vi "исходные пределы.vi"() -> ()   [LabVIEW 2013]
panel:
  in  "X1":dbl[][](array[numeric])=[[0.1, 20.0], [0.5, 200.0], [1.0, 200.0], [3.0, 2000.0], [5.0, 2000.0], [10.0, 2000.0], [15.0, 10000.0], [20.0, 10000.0], [25.0, 10000.0], [30.0, 10000.0], [35.0, 10000.0], [40.0, 10000.0], [45.0, 10000.0], [50.0, 10000.0], [55.0, 10000.0], [60.0, 10000.0], [65.0, 10000.0], [70.0, 10000.0], [75.0, 10000.0], [80.0, 10000.0], [85.0, 10000.0], [90.0, 10000.0], [95.0, 10000.0], [100.0, 10000.0]] format="%0.3f"
  in  "X2":dbl[][](array[numeric])=[[0.1, 20.0], [0.5, 200.0], [1.0, 200.0], [3.0, 200.0], [5.0, 2000.0], [10.0, 2000.0], [15.0, 2000.0], [20.0, 2000.0], [25.0, 2000.0], [30.0, 2000.0], [35.0, 2000.0], [40.0, 2000.0], [45.0, 10000.0], [50.0, 10000.0], [55.0, 10000.0], [60.0, 10000.0], [65.0, 10000.0], [70.0, 10000.0], [75.0, 10000.0], [80.0, 10000.0], [85.0, 10000.0], [90.0, 10000.0], [95.0, 10000.0], [100.0, 10000.0]] format="%0.3f"
  in  "X3":dbl[][](array[numeric])=[[0.1, 20.0], [0.5, 20.0], [1.0, 200.0], [3.0, 200.0], [5.0, 200.0], [10.0, 2000.0], [15.0, 2000.0], [20.0, 2000.0], [25.0, 2000.0], [30.0, 2000.0], [35.0, 2000.0], [40.0, 2000.0], [45.0, 2000.0], [50.0, 2000.0], [55.0, 2000.0], [60.0, 2000.0], [65.0, 2000.0], [70.0, 2000.0], [75.0, 2000.0], [80.0, 2000.0], [85.0, 2000.0], [90.0, 2000.0], [95.0, 2000.0], [100.0, 2000.0]] format="%0.3f"
  in  "X6":dbl[][](array[numeric])=[[0.1, 2.0], [0.5, 20.0], [1.0, 20.0], [3.0, 20.0], [5.0, 200.0], [10.0, 200.0], [15.0, 200.0], [20.0, 200.0], [25.0, 200.0], [30.0, 200.0], [35.0, 200.0], [40.0, 200.0], [45.0, 2000.0], [50.0, 2000.0], [55.0, 2000.0], [60.0, 2000.0], [65.0, 2000.0], [70.0, 2000.0], [75.0, 2000.0], [80.0, 2000.0], [85.0, 2000.0], [90.0, 2000.0], [95.0, 2000.0], [100.0, 2000.0]] format="%0.3f"
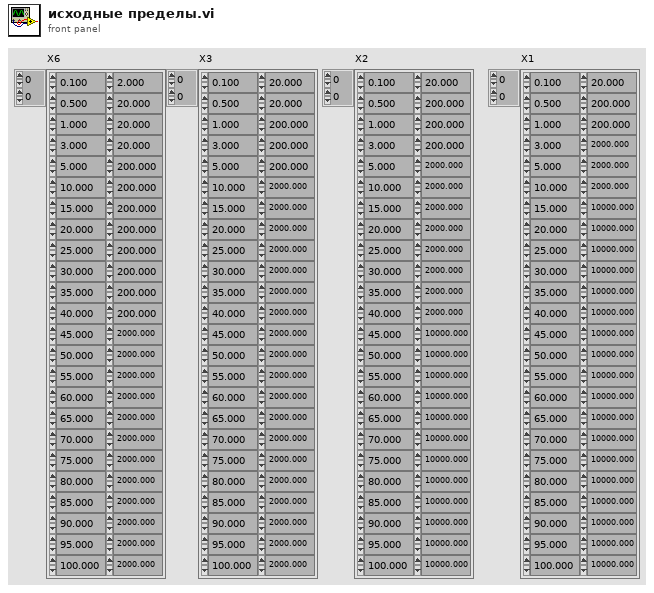
[diagram p1: front panel]
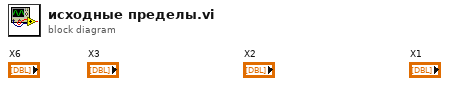
[diagram p0: block diagram]
diagram:
